vi "Controller To Device.vi"(0 "Notifier":refnum<notifier>, 1 "Message queue":refnum<queue>, 2 "Message Priority ?":bool, 3 "Message":string, 4 "Data":variant, 5 "entrée d'erreur":errorcluster caption="entrée d'erreur (pas d'erreur)") -> (14 "Dup Message queue":refnum<queue>, 15 "notification":variant, 19 "sortie d'erreur":errorcluster)   [LabVIEW 2013]
doc: "Ce VI rentre un message avec une donnée dans une pile et attend en retour la confirmation de la réception de ce message via un notifier\nOn y trouve donc en Entrée\n- le notifier de confirmation\n- la pile (queue) fesant l'objet du message\n- le message (chaine de caractère)\n- la donnée du type variant\n- un booléen indiquant si le message est prioritaire => vrai : le message est mis au début de la pile. Faux : le message est mis à la fin de la pile\n- le cordont d'erreur.\n\nEn sortie :\n- la pile incrémenté\n- la donnée lié à la notification (variant)\n- le cordont d'erreur de sortie"
uses:
  Lib QMH/Message Cluster.ctl
  Lib QMH/MessageQueues.lvlib
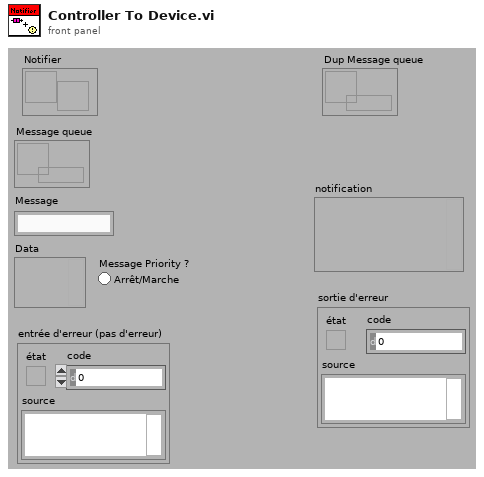
[diagram p1: front panel]
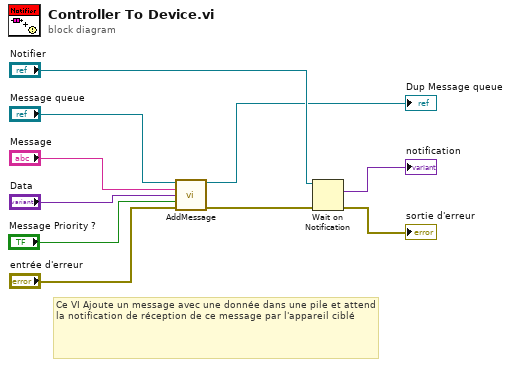
[diagram p0: block diagram]
diagram:
  # "Ce VI Ajoute un message avec une donnée dans une pile et attend la notification de réception de ce message par l'appareil ciblé"
  n1 = call "AddMessage.vi"("Message queue"="Message queue", "Message"="Message", "Data"="Data", "Message Priority ?"="Message Priority ?", "entrée d'erreur (pas d'erreur)"="entrée d'erreur") -> ("Dup Message queue"=→"Dup Message queue":refnum<queue>, "error out"=w6:errorcluster)  [unwired: 9 in]
  n2 = Wait on Notification(notifier="Notifier", error in (no error)=w6) -> (notification=→"notification":variant, error out=→"sortie d'erreur":errorcluster)  [unwired: 2 in, 2 out]
